vi "Flatten Value.vi"(8 "Error In":errorcluster, 11 "StringArray In":refnum<class "1D String.lvclass">) -> (0 "Error Out":errorcluster, 1 "Value":string, 3 "StringArray Out":refnum<class "1D String.lvclass">)   [LabVIEW 2020, in "NI_VIAnCFGDataStructure.lvlib" / "1D String.lvclass"]
uses:
  <vilib>/addons/analyzer/VIAnCFGDataStructure/Data Types/String Array/1D String.lvclass
  <vilib>/addons/analyzer/VIAnCFGDataStructure/Data Types/String Array/1D String.lvclass/1D String.ctl
  <vilib>/addons/analyzer/VIAnCFGDataStructure/Tree Manager/API/Generate Hash.vi
  <vilib>/addons/analyzer/VIAnCFGDataStructure/Tree Manager/Tree.lvclass
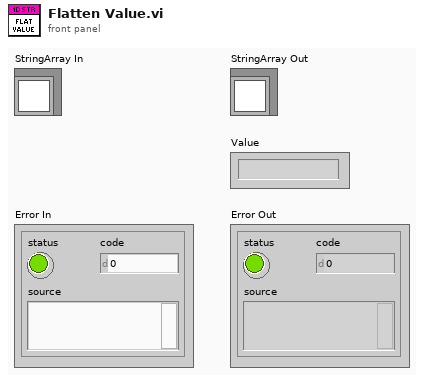
[diagram p1: front panel]
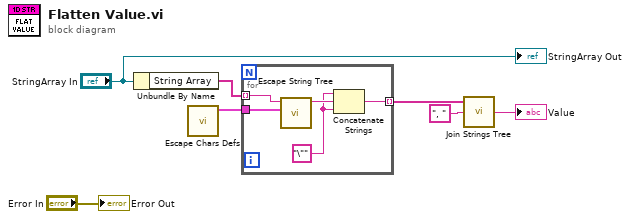
[diagram p0: block diagram]
diagram:
  n1 = Unbundle By Name("StringArray In") -> ("String Array"=w4:string[])
  n2 = call <vilib>:"Escape Chars Defs.vi"() -> ("Escapes"=w5:cluster{"String":string, "Escape":string}[])  [unwired: 11 in]
  n3 = for {
    tunnel: w4 -> [w11] mode=indexing
    tunnel: w5 -> [w12]
    tunnel: [w8] -> w2 mode=indexing
    w9 = "\"" ("string")
    n4 = call <vilib>:"Escape String Tree.vi"("Escapes"=w12, "String In"=w11) -> ("String Out"=w10:string)  [unwired: 9 in]
    n5 = Concatenate Strings(w9, w10, w9) -> (w8:string)
  }
  n6 = call <vilib>:"Join Strings Tree.vi"("Separator (,)"=", ", "Strings In"=w2) -> ("String"=→"Value":string)  [unwired: 1 in]
  "StringArray Out" <- "StringArray In"
  "Error Out" <- "Error In"
